vi "FF_SetViaPts.vi"(8 "error in (no error)":errorcluster, 10 "Path via Points":dbl[][](array[numeric]), 11 "Force Field Controller in":refnum<class "ForceField.lvclass">) -> (0 "error out":errorcluster, 3 "Force Field Controller out":refnum<class "ForceField.lvclass">)   [LabVIEW 2016, in "ForceField.lvclass"]
uses:
  ForceField.lvclass
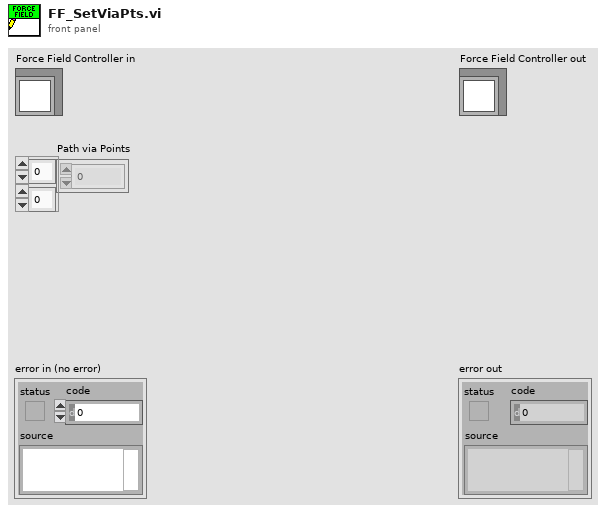
[diagram p1: front panel]
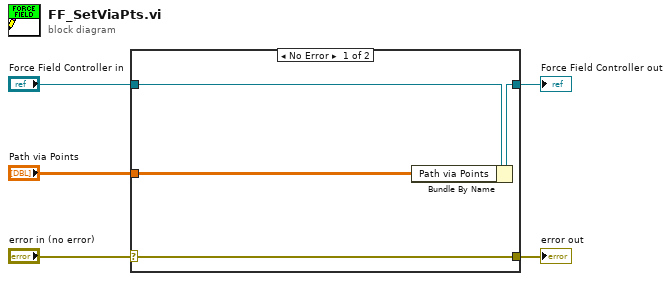
[diagram p0: block diagram]
diagram:
  n1 = case shown="No Error" "error in (no error)" {
    selector: "error in (no error)" -> [w9 w10]
    tunnel: [w9 w10] -> w4
    tunnel: [w7 w11] -> w2
    tunnel: "Force Field Controller in" -> [w8 w11]
    tunnel: "Path via Points" -> [w6 _]
    frame No Error {
      n2 = Bundle By Name(cluster=w8, "Path via Points"=w6) -> (w7:refnum<class "ForceField.lvclass">)
    }
    frame Error {
    }
  }
  "error out" <- w4
  "Force Field Controller out" <- w2
